vi "Phase to Matrix.vi"(9 "Target Retrieved \nPhase":path=path "C:/Users/Green Beret/Documents/Visual Studio 2012/Projects/LightPipes/LightPipes/lp12src/LabView/images/target_retrieved_phase.gpl", 10 "num rows":i32=256, 11 "field":T1) -> (2 "Phase":dbl[][](array[numeric]) format="%0.3f", 3 "field out":T1)   [LabVIEW 2012, in "LightPipes.lvlib"]
uses:
  Lightpipes.lvlib
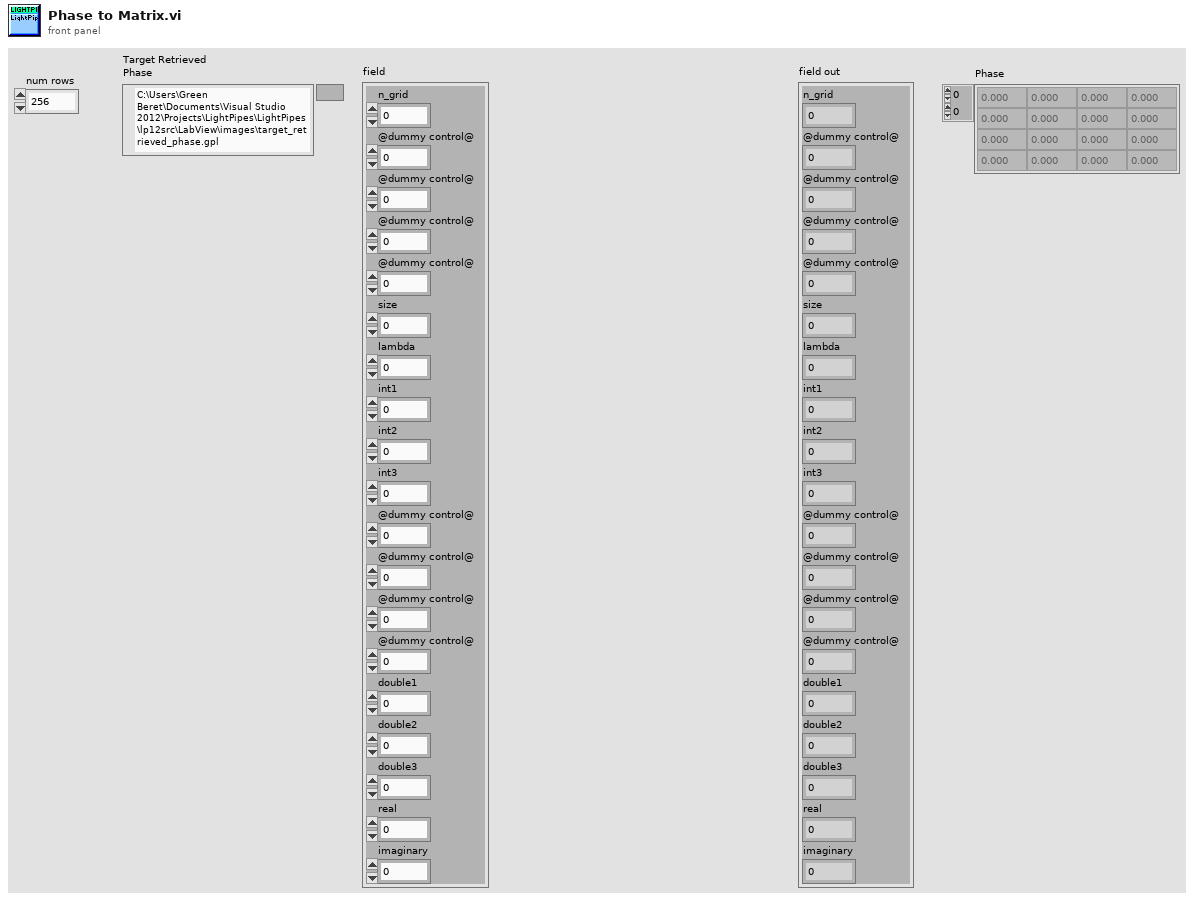
[diagram p1: front panel]
types:
  T1 = cluster{"n_grid":i32, "@dummy control@":i8, "@dummy control@":i8, "@dummy control@":i8, "@dummy control@":i8, "size":dbl, "lambda":dbl, "int1":i32, "int2":i32, "int3":i32, "@dummy control@":i8, "@dummy control@":i8, "@dummy control@":i8, "@dummy control@":i8, "double1":dbl, "double2":dbl, "double3":dbl, "real":u32, "imaginary":u32}
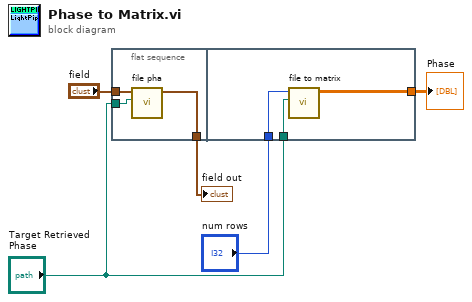
[diagram p0: block diagram]
diagram:
  n1 = flat-sequence {
    tunnel: "field" -> [w8]
    tunnel: [w7] -> w4
    tunnel: "Target Retrieved \nPhase" -> [w6]
    tunnel: "num rows" -> [w11]
    tunnel: "Target Retrieved \nPhase" -> [w10]
    tunnel: [w9] -> w1
    frame #0 {
      n2 = call "file pha.vi"("Path in"=w6, "field"=w8) -> ("field out"=w7:T1)  [unwired: 8 in, 1 out]
    }
    frame #1 {
      n3 = call "file to matrix.vi"("File Path"=w10, "number of rows (all:-1)"=w11) -> ("all rows"=w9:dbl[][])  [unwired: 9 in]
    }
  }
  "field out" <- w4
  "Phase" <- w1
